vi "Verify Calibration.vi"(8 "error in (no error)":errorcluster, 11 "Configuration in":refnum<class "Configuration.lvclass">) -> (0 "error out":errorcluster, 3 "Configuration out":refnum<class "Configuration.lvclass">)   [LabVIEW 2018, in "Configuration.lvlib" / "Configuration.lvclass"]
doc: "Check config.ini file for calibration due dates for the selected device. \n\nIf cal is overdue, produce an error message\nIf cal is due within 30 days, pop -up a dialog notifying operator\nIf cal is not due for more than 30 days, return no error or dialog"
uses:
  Configuration.lvclass
  Configuration.lvclass/Configuration.ctl
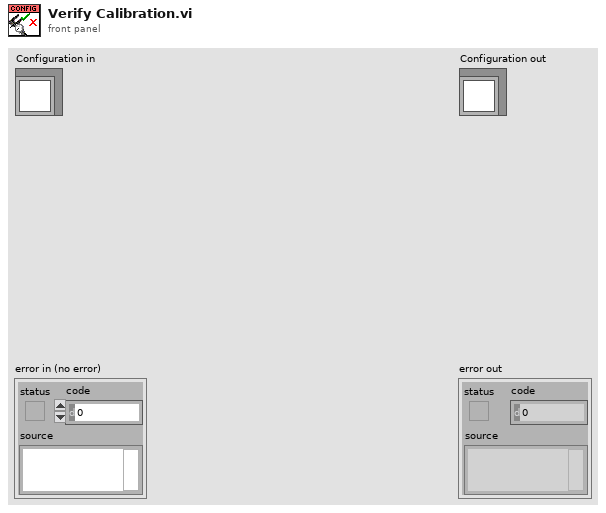
[diagram p1: front panel]
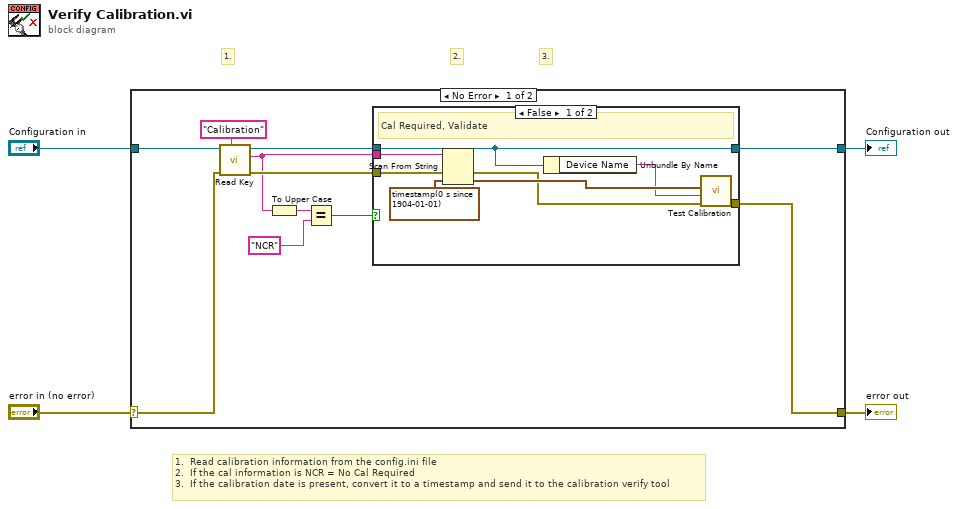
[diagram p0: block diagram]
diagram:
  # "1.  Read calibration information from the config.ini file\n2.  If the cal information is NCR = No Cal Required\n3.  If the calibration date is present, convert it to a timestamp and send it to the calibration verify tool"
  # "3."
  # "2."
  # "1."
  n1 = case shown="No Error" "error in (no error)" {
    selector: "error in (no error)" -> [w13 w27]
    tunnel: [w11 w27] -> w3
    tunnel: [w6 w26] -> w1
    tunnel: "Configuration in" -> [w15 w26]
    frame No Error {
      n2 = call "Read Key.vi"("Key:"="Calibration", "error in"=w13, "Configuration in"=w15) -> ("error out"=w12:errorcluster, "Value"=w9:string, "Configuration out"=w10:refnum<class "Configuration.lvclass">)  [unwired: 6 in]
      n3 = To Upper Case(1:w9) -> (0:w8:string)
      n4 = Equal?(x=w8, y="NCR") -> (x = y?=w5:bool)
      n5 = case shown="False" w5 {
        tunnel: w12 -> [w23 w24]
        tunnel: [w19 w24] -> w11
        tunnel: w10 -> [w16 w25]
        tunnel: w9 -> [w17 _]
        tunnel: [w16 w25] -> w6
        frame False {
          # "Cal Required, Validate"
          n6 = Scan From String(input string=w17, error in=w23, default 1=timestamp(0 s since 1904-01-01) ("default value 1")) -> (error out=w21:errorcluster, output 1=w22:timestamp)  [unwired: 2 in, 2 out]
          n7 = Unbundle By Name(w16) -> ("Device Name"=w18:string)
          n8 = call "Test Calibration.vi"("error in"=w21, "Device"=w18, "Cal Data"=w22) -> ("error out"=w19:errorcluster)  [unwired: 8 in]
        }
        frame True {
          # "No Calibration Required"
        }
      }
    }
    frame Error {
    }
  }
  "error out" <- w3
  "Configuration out" <- w1
